vi "instrumentProperties_channels.vi"(8 "error in (no error)":errorcluster, 11 "Thorlabs_OSA200_64 in":refnum<class "OSA200.lvclass">) -> (0 "error out":errorcluster, 1 "channel properties":T2[](array[typedef]), 2 "channels nr":i32, 3 "Thorlabs_OSA200_64 out":refnum<class "OSA200.lvclass">, 4 "channelType_spectrum":T1, 5 "channel DUT (index)":i32)   [LabVIEW 2010, in "OSA200.lvclass"]
uses:
  OSA200.lvclass
  _misc/Thorlabs_FTS_misc.llb/channel_propertiesGen.ctl
  _misc/Thorlabs_FTS_misc.llb/detector_sort.ctl
  _misc/Thorlabs_FTS_misc.llb/channelType_spectrum.ctl
  OSA.lvclass
  OSA20X_misc.lvlib
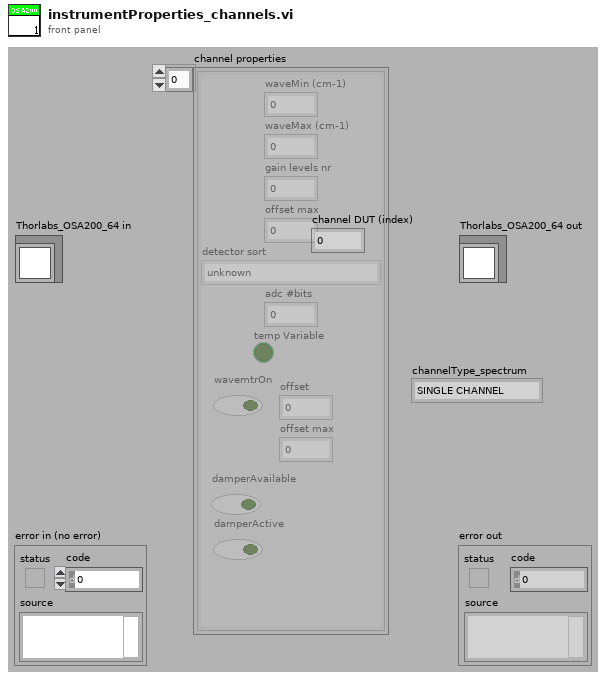
[diagram p1: front panel]
types:
  T1 = typedef "OSA20X_misc.lvlib/channelType_spectrum.ctl" = enum16{"SINGLE CHANNEL", "STICHED"}
  T2 = typedef "OSA20X_misc.lvlib/channel_propertiesGen.ctl" = cluster{"waveMin (cm-1)":sgl, "waveMax (cm-1)":sgl, "gain levels nr":u16, "offset max":u16, "detector sort":T3, "adc #bits":u16, "temp Variable":bool, "wavemtrOn":bool, "offset":i32, "offset max":u16, "damperAvailable":bool, "damperActive":bool}
  T3 = typedef "OSA20X_misc.lvlib/detector_sort.ctl" = enum16{"unknown", "Silicon", "Silicon PIN", "Silicon MPPC", "InGaAs", "InGaAs ext low", "InGaAs ext high", "InAs", "InAsSb", "InSb", "MCT", "other", "other2", "other3"}
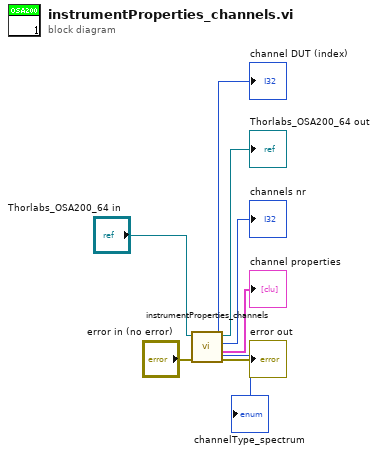
[diagram p0: block diagram]
diagram:
  n1 = call-parent "instrumentProperties_channels.vi"("error in (no error)"="error in (no error)", "Thorlabs_OSA_64 in"="Thorlabs_OSA200_64 in") -> ("error out"=→"error out":errorcluster, "channel properties"=→"channel properties":T2[], "channels nr"=→"channels nr":i32, "Thorlabs_OSA_64 out"=→"Thorlabs_OSA200_64 out":refnum<class "OSA200.lvclass">, "spectrum channel type"=→"channelType_spectrum":T1, "channel DUT (index)"=→"channel DUT (index)":i32)  [unwired: 4 in]
